vi "Start SubComponent.vi"(5 "Component ID":u8, 7 "FPGA Interface":refnum<class "FPGA Interface.lvclass">, 8 "error in (no error)":errorcluster, 11 "Bus Controller in":refnum<class "Bus Controller.lvclass">) -> (0 "error out":errorcluster, 3 "Bus Controller out":refnum<class "Bus Controller.lvclass">)   [LabVIEW 2020, in "BCI-1553 API.lvlib" / "Bus Controller.lvclass"]
doc: "Ensures that the Bus Controller is enabled and starts its operation."
uses:
  Bus Controller.lvclass
  Dependencies/FPGA Interface/FPGA Interface.lvclass
panel:
  out "Master":u16 format="%04x"
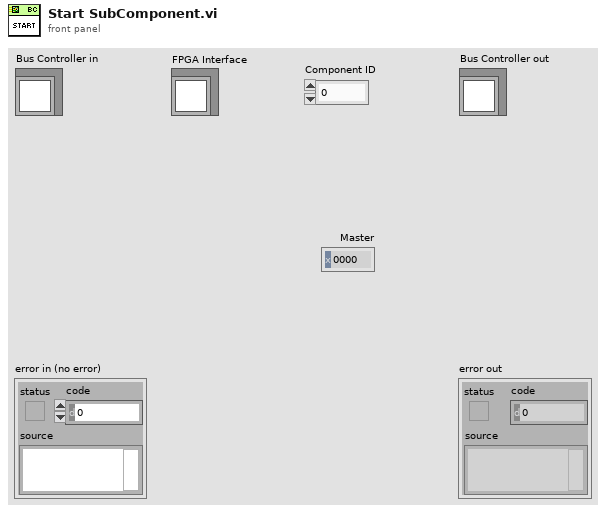
[diagram p1: front panel]
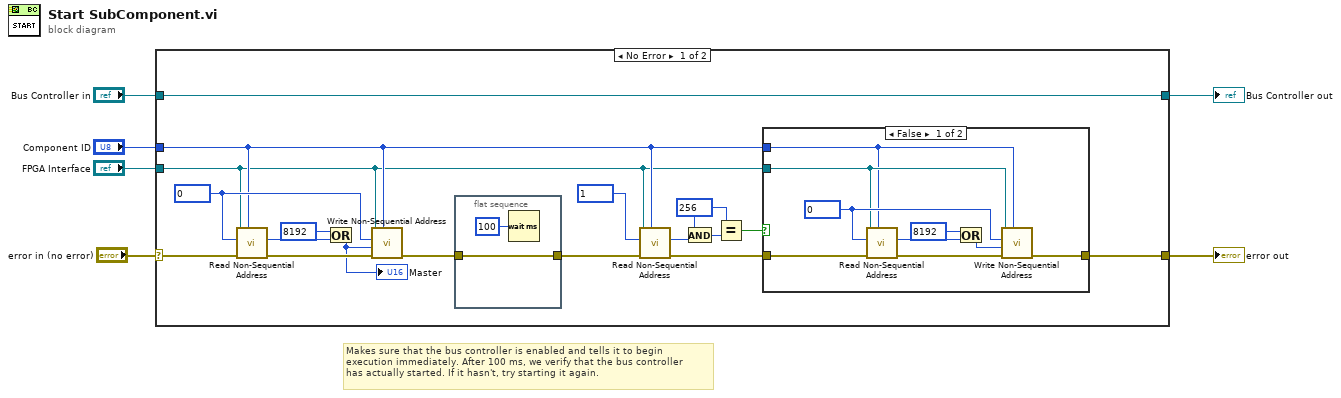
[diagram p0: block diagram]
diagram:
  # "Makes sure that the bus controller is enabled and tells it to begin\nexecution immediately. After 100 ms, we verify that the bus controller\nhas actually started. If it hasn't, try starting it again."
  n1 = case shown="No Error" "error in (no error)" {
    selector: "error in (no error)" -> [w24 w38]
    tunnel: [w9 w38] -> w5
    tunnel: "Bus Controller in" -> [w20 w37]
    tunnel: "FPGA Interface" -> [w7 _]
    tunnel: "Component ID" -> [w8 _]
    tunnel: [w20 w37] -> w1
    frame No Error {
      w12 = u16 256 ("Address")
      w19 = u16 0 ("Address")
      n2 = call-dynamic "Read Non-Sequential Address.vi"("Target IC (1-8)"=w8, "error in (no error)"=w24, "Address"=w19, "FPGA Interface in"=w7) -> ("error out"=w23:errorcluster, "Data"=w21:u16)  [unwired: 6 in]
      n3 = Or(x=u16 8192 ("Address"), y=w21) -> (x .or. y?=w18:u16)
      "Master" <- w18
      n4 = call-dynamic "Write Non-Sequential Address.vi"("Target IC (1-8)"=w8, "error in (no error)"=w23, "Data"=w18, "Address"=w19, "FPGA Interface in"=w7) -> ("error out"=w17:errorcluster)  [unwired: 6 in]
      n5 = flat-sequence {
        tunnel: w17 -> [w35]
        tunnel: [w35] -> w15
        frame #0 {
          n6 = Wait (ms)(milliseconds to wait=u32 100) -> ()  [unwired: 1 out]
        }
      }
      n7 = call-dynamic "Read Non-Sequential Address.vi"("Target IC (1-8)"=w8, "error in (no error)"=w15, "Address"=u16 1, "FPGA Interface in"=w7) -> ("error out"=w11:errorcluster, "Data"=w14:u16)  [unwired: 6 in]
      n8 = And(x=w12, y=w14) -> (x .and. y?=w13:u16)
      n9 = Equal?(x=w12, y=w13) -> (x = y?=w10:bool)
      n10 = case shown="False" w10 {
        tunnel: w11 -> [w28 w34]
        tunnel: [w27 w34] -> w9
        tunnel: w8 -> [w25 _]
        tunnel: w7 -> [w26 _]
        frame False {
          w32 = u16 0 ("Address")
          n11 = call-dynamic "Read Non-Sequential Address.vi"("Target IC (1-8)"=w25, "error in (no error)"=w28, "Address"=w32, "FPGA Interface in"=w26) -> ("error out"=w29:errorcluster, "Data"=w31:u16)  [unwired: 6 in]
          n12 = Or(x=u16 8192 ("Address"), y=w31) -> (x .or. y?=w33:u16)
          n13 = call-dynamic "Write Non-Sequential Address.vi"("Target IC (1-8)"=w25, "error in (no error)"=w29, "Data"=w33, "Address"=w32, "FPGA Interface in"=w26) -> ("error out"=w27:errorcluster)  [unwired: 6 in]
        }
        frame True {
        }
      }
    }
    frame Error {
    }
  }
  "error out" <- w5
  "Bus Controller out" <- w1
